vi "labSelector.vi"() -> (3 "Numeric":dbl)   [LabVIEW 2014]
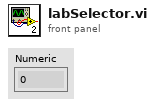
[diagram p1: front panel]
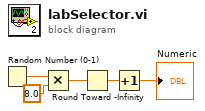
[diagram p0: block diagram]
diagram:
  n1 = Random Number (0-1)() -> (number: 0 to 1=w5:dbl)
  n2 = Multiply(x=w5, y=8.0) -> (x*y=w3:dbl)
  n3 = Round Toward -Infinity(1:w3) -> (0:w2:dbl)
  n4 = Increment(x=w2) -> (x+1=→"Numeric":dbl)
